vi "Absolute Angle Difference (array).vi"(7 "angle units":T1 items=["radian in, radian out", "radian in, degree out", "degree in, degree out", "degree in, radian out"], 10 "Angle 2":dbl[](array[numeric]), 11 "Angle 1":dbl[](array[numeric])) -> (0 "error":i32, 3 "Absolute Angle Difference":dbl[](array[numeric]))   [LabVIEW 2017, in "NI_AAL_Angle.lvlib"]
doc: "Calculates the absolute difference between two input angles or multiple pairs of input angles.\n\nWire data to any of the angle inputs to determine the polymorphic instance to use or manually select the instance."
uses:
  <vilib>/Analysis/NI_AAL_Angle.lvlib
  <vilib>/Analysis/coordinate.llb/Angle Units.ctl
  <vilib>/Analysis/coordinate.llb/Angle Range (Degree).ctl
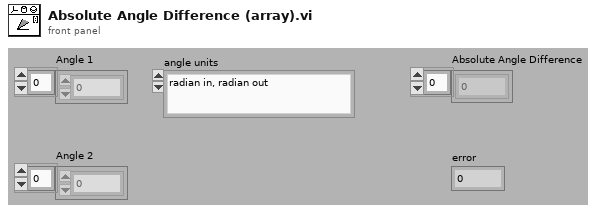
[diagram p1: front panel]
types:
  T1 = typedef "NI_AAL_Angle.lvlib/Angle Units.ctl" = i32
  T2 = typedef "NI_AAL_Angle.lvlib/Angle Range (Degree).ctl" = u16
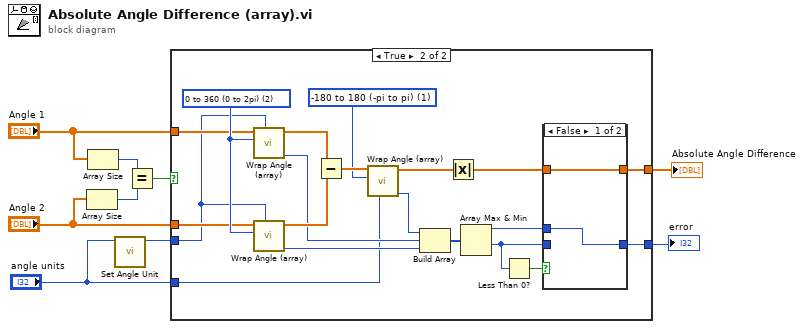
[diagram p0: block diagram]
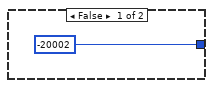
[diagram p2: hidden frame]
diagram:
  n1 = Array Size(array="Angle 2") -> (size(s)=w5:i32)
  n2 = Array Size(array="Angle 1") -> (size(s)=w4:i32)
  n3 = call <vilib>:"Set Angle Unit.vi"("angle units in"="angle units") -> ("angle units out"=w2:T1)  [unwired: 10 in]
  n4 = Equal?(x=w4, y=w5) -> (x = y?=w3:bool)
  n5 = case shown="True" w3 {
    tunnel: [-20002 w17] -> w9
    tunnel: [_ w16] -> w8
    tunnel: "Angle 1" -> [_ w15]
    tunnel: "Angle 2" -> [_ w14]
    tunnel: w2 -> [_ w11]
    tunnel: "angle units" -> [_ w12]
    frame False {
    }
    frame True {
      w13 = T2 1 items=["none", "-180 to 180 (-pi to pi)", "0 to 360 (0 to 2pi)"] ("angle range")
      w30 = T2 2 items=["none", "-180 to 180 (-pi to pi)", "0 to 360 (0 to 2pi)"] ("angle range")
      n6 = call <vilib>:"Wrap Angle (array).vi"("angle units"=w11, "angle range"=w30, "Angle In"=w15) -> ("error"=w25:i32, "Angle Out"=w29:dbl[])  [unwired: 7 in]
      n7 = call <vilib>:"Wrap Angle (array).vi"("angle units"=w11, "angle range"=w30, "Angle In"=w14) -> ("error"=w24:i32, "Angle Out"=w28:dbl[])  [unwired: 7 in]
      n8 = Subtract(x=w29, y=w28) -> (x-y=w27:dbl[])
      n9 = call <vilib>:"Wrap Angle (array).vi"("angle units"=w12, "angle range"=w13, "Angle In"=w27) -> ("error"=w23:i32, "Angle Out"=w26:dbl[])  [unwired: 7 in]
      n10 = Build Array(w23, w25, w24) -> (w22:i32[])
      n11 = Absolute Value(x=w26) -> (abs(x)=w20:dbl[])
      n12 = Array Max & Min(array=w22) -> (max value=w18:i32, min value=w19:i32)  [unwired: 2 out]
      n13 = Less Than 0?(x=w19) -> (x < 0?=w21:bool)
      n14 = case shown="False" w21 {
        tunnel: w20 -> [w32 _]
        tunnel: [w32 _] -> w16
        tunnel: w19 -> [_ w33]
        tunnel: [w31 w33] -> w17
        tunnel: w18 -> [w31 _]
        frame False {
        }
        frame True {
        }
      }
    }
  }
  "Absolute Angle Difference" <- w8
  "error" <- w9
